vi "AllenBradlenLightSensor-AnalogInput.vi"() -> ()   [LabVIEW 2020]
doc: "Analog Input Example\n\nThis example will read voltages from an analog channel and display it on a chart. It will also display the average voltage over time. \n\nThe values for Average Bits and Samples Per Second on the front panel can be set while the VI is running.\n\nThis example expects a USB cable connected from your development PC to the Type B USB Jack (next to the power input) on the roboRIO."
uses:
  <vilib>/Rock Robotics/SystemInterfaces/AI/FPGA_AIChannel.ctl
  <vilib>/Rock Robotics/WPI/Utilities/WPI_GetSetVariantRefNum.vi
panel:
  in  "Analog Channel":T1
  out "error out 2":errorcluster
  out "error out":errorcluster
  out "Voltage Display":cluster{"Value":dbl, "Voltage":dbl}(graph)
  out "Average Voltage":dbl
  out "Voltage":dbl
  # "Set this input before running."
  # "These can be set while running."
  # "This chart displays the voltage and average voltage over time."
  # "This shows wiring for a typical analog input using a potentiometer.  In this case the potentiometer is being powered with 5 volts, and the Signal returned will vary from 0 to 5 volts"
  # "potentiometer"
  # "Gnd"
  # "S"
  # "V"
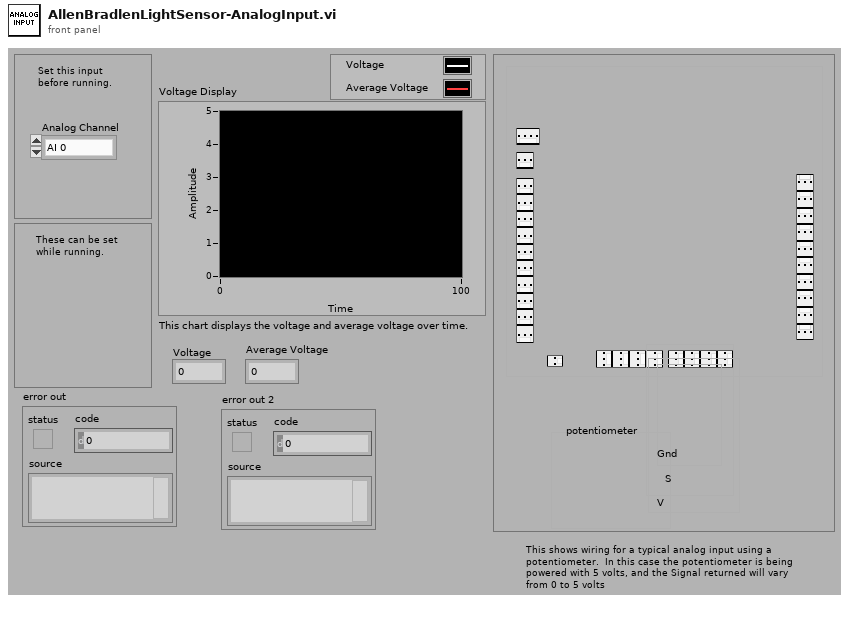
[diagram p1: front panel]
types:
  T1 = typedef "FPGA_AIChannel.ctl" = enum8{"AI 0", "AI 1", "AI 2", "AI 3", "AI MXP 0", "AI MXP 1", "AI MXP 2", "AI MXP 3", "Invalid"}
  T2 = typedef "WPI_AnalogChannelDevRef.ctl" = cluster{"DevStatus":errorcluster, "Analog Channel":T1}
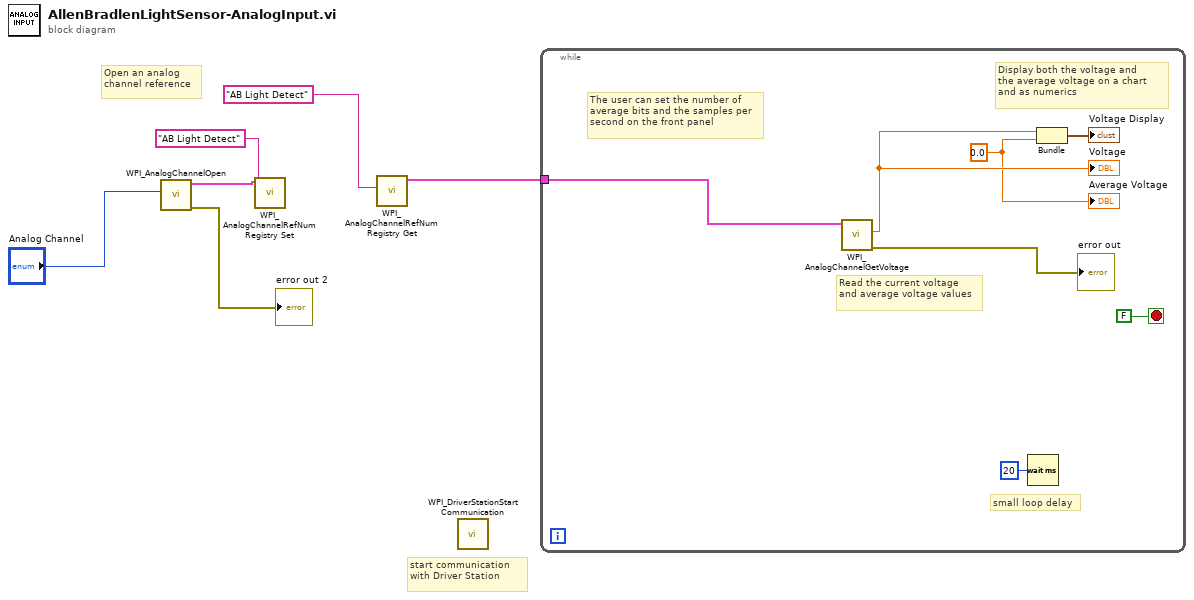
[diagram p0: block diagram]
diagram:
  # "start communication with Driver Station"
  # "Open an analog channel reference"
  n1 = call <vilib>:"WPI_AnalogChannelOpen.vi"("Analog Channel"="Analog Channel") -> ("error out"=→"error out 2":errorcluster, "AIDeviceRef"=w2:T2)  [unwired: 9 in]
  n2 = call <vilib>:"WPI_AnalogChannelRefNum Registry Set.vi"("refnum name"="AB Light Detect", "AIDeviceRef"=w2) -> ()  [unwired: 8 in, 2 out]
  n3 = call <vilib>:"WPI_AnalogChannelRefNum Registry Get.vi"("refnum name"="AB Light Detect") -> ("AIDeviceRef"=w4:T2)  [unwired: 9 in, 1 out]
  n4 = call <vilib>:"WPI_DriverStationStart Communication.vi"() -> ()  [unwired: 3 in, 9 out]
  n5 = while {
    tunnel: w4 -> [w11]
    stop <- FALSE stop-if-true
    w7 = 0.0
    # "small loop delay"
    # "Read the current voltage\nand average voltage values"
    # "Display both the voltage and\nthe average voltage on a chart\nand as numerics"
    # "The user can set the number of \naverage bits and the samples per\nsecond on the front panel"
    n6 = call <vilib>:"WPI_AnalogChannelGetVoltage.vi"("AIDeviceRef"=w11) -> ("error out"=→"error out":errorcluster, "Voltage"=w13:dbl)  [unwired: 1 in, 8 out]
    "Voltage" <- w13
    n7 = Wait (ms)(milliseconds to wait=u32 20) -> ()  [unwired: 1 out]
    n8 = Bundle("Voltage"=w13, w7) -> (→"Voltage Display":cluster{"Voltage":dbl, dbl})  [unwired: 1 out]
    "Average Voltage" <- w7
  }
